vi "ScannerMain.vi"() -> ()   [LabVIEW 2012]
uses:
  Strict Type Def - Scan Parameters Cluster.ctl
  Strict Type Def - Optimize Parameters Cluster.ctl
  Rabi Window Parameters.ctl
  ESR Window Parameters.ctl
  Spin Echo Window Parameters.ctl
  Window Parameters-CPMG.ctl
  SaveContrastOptions.ctl
  Window Parameters-XY4.ctl
  States.ctl
  Global Vars.vi
  Channels.vi
panel:
  in  "Program":T1(tab)=enum."CPMG"
  in  "Z Voltage":dbl min=-10.0 max=10.0 step=0.1
  in  "Continuous":bool
  in  "Green Laser (low-T)":bool caption="Scan"
  in  "Microwave":bool caption="Scan"
  in  "Green Laser":bool=TRUE caption="Scan"
  out "Counts Intensity Graph":i32[][](graph)
  in  "Scan Parameters":T2={"X Max"=1.5, "X Min"=-1.5, "X Step"=0.02, "Y Max"=1.5, "Y Min"=-1.5, "Y Step"=0.02, "Dwell Time (ms) "=1} {"Dwell Time (ms)" min=0; "Y Step" min=0.0; "X Step" min=0.0}
  in  "Optimize":bool
  in  "Scan":bool
  in  "Count":bool caption="Optimize"
  out "Counts Chart":u32(graph)=11280
  out "Counts/s":i32=11280
  in  "Optimize Parameters":T3={"Volt Step"={"X"=0.005, "Y"=0.005, "Z"=0.0}, "Num Iterations"=5, "Dwell Time (ms)"=25, "Volts Range"={"X"=0.05, "Y"=0.05, "Z"=0.0}, "Method"={"X"=enum."Max", "Y"=enum."Max", "Z"=enum."Max"}} {"Volts Range"."Z" min=0.0; "Volts Range"."Y" min=0.0; "Volts Range"."X" min=0.0; "Dwell Time (ms)" min=0; "Num Iterations" min=1 step=1; "Volt Step"."Z" min=0.0; "Volt Step"."Y" min=1e-06; "Volt Step"."X" min=1e-06}
  in  "ESR":bool caption="Scan"
  in  "ESR spectrum spreadsheet":path=path "C:/experiment/data/may_15_2012/SIL1_NV1_pippin_uW_off"
  in  "Save ESR spectrum data":bool
  in  "ESR spectrum graph":path=path "C:/experiment/data/may_15_2012/SIL1_NV1_pippin_uW_off"
  in  "Save ESR spectrum graph":bool
  out "Avg ESR spectrum":cluster{"Y":dbl[], "Y":dbl[]}[](graph)=[{"Y"=[2.82, 2.8202499999999997, 2.8205, 2.82075, 2.8209999999999997, 2.82125, 2.8215, 2.8217499999999998, 2.822, 2.82225, 2.8225, 2.8227499999999996, 2.823, 2.82325, 2.8234999999999997, 2.82375, 2.824, 2.8242499999999997, 2.8245, 2.82475, 2.8249999999999997, 2.82525, 2.8255, 2.8257499999999998, 2.8259999999999996, 2.82625, 2.8265, 2.8267499999999997, 2.827, 2.82725, 2.8274999999999997, 2.82775, 2.828, 2.8282499999999997, 2.8285, 2.82875, 2.8289999999999997, 2.82925, 2.8295, 2.8297499999999998, 2.83, 2.83025, 2.8305, 2.8307499999999997, 2.831, 2.83125, 2.8314999999999997, 2.83175, 2.832, 2.8322499999999997, 2.8325, 2.83275, 2.8329999999999997, 2.83325, 2.8335, 2.8337499999999998, 2.8339999999999996, 2.83425, 2.8345, 2.8347499999999997, 2.835, 2.83525, 2.8354999999999997, 2.83575, 2.836, 2.8362499999999997, 2.8365, 2.83675, 2.8369999999999997, 2.83725, 2.8375, 2.8377499999999998, 2.838, 2.83825, 2.8385, 2.8387499999999997, 2.839, 2.83925, 2.8394999999999997, 2.83975, 2.84], "Y"=[256.4611111111111, 260.3277777777778, 260.22777777777776, 259.8, 256.4, 257.15, 255.9388888888889, 257.1111111111111, 259.4166666666667, 256.89444444444445, 256.6111111111111, 257.1333333333333, 258.4611111111111, 257.9222222222222, 256.1333333333333, 256.74444444444447, 255.5388888888889, 257.95, 255.46666666666667, 254.41666666666666, 255.3, 253.4611111111111, 253.63888888888889, 255.43333333333334, 252.68333333333334, 250.01111111111112, 248.7722222222222, 249.03333333333333, 247.25, 249.34444444444443, 248.07222222222222, 248.8, 250.05, 251.64444444444445, 250.7, 252.01111111111112, 248.62222222222223, 251.03333333333333, 248.46666666666667, 249.4388888888889, 249.24444444444444, 248.97222222222223, 250.43333333333334, 250.25, 252.8388888888889, 253.66666666666666, 253.85555555555555, 253.97222222222223, 257.25, 256.47777777777776, 257.18333333333334, 257.6722222222222, 257.19444444444446, 257.81111111111113, 257.4555555555556, 256.5444444444444, 260.69444444444446, 257.3722222222222, 258.3, 259.3722222222222, 258.1611111111111, 259.81666666666666, 258.8333333333333, 257.68333333333334, 255.70555555555555, 260.22222222222223, 256.3777777777778, 258.59444444444443, 260.6666666666667, 257.40555555555557, 257.5833333333333, 259.4555555555556, 259.5777777777778, 259.68888888888887, 258.97222222222223, 258.35, 258.84444444444443, 258.34444444444443, 260.6333333333333, 256.51666666666665, 259.43333333333334]}]
  out "Counts vs. frequency":i32[][](graph)
  in  "# freq points":i32=81
  in  "MW start freq (GHz)":dbl=2.82
  in  "MW stop freq (GHz)":dbl=2.84
  in  "# scans before track":i32=20
  in  "#scan iterations":i32=20
  in  "ESR Parameters":T4={"Window 1 time (s)"=0.005, "Window 2 time (s)"=5e-06, "Window 3 time (s) "=0.02, "Window 4 time (s)"=5e-07, "Window 4 channels"=[TRUE, FALSE, FALSE, TRUE], "Window 3 channels"=[TRUE, FALSE, TRUE, TRUE], "Window 2 channels"=[TRUE, FALSE, FALSE, TRUE], "Window 1 channels"=[TRUE, TRUE, FALSE, TRUE], "Path to ESR Burner"=path "C:/Users/Loncar/Desktop/ESR VIs - Srujan/Sam Kim/PB/ESRFreq.exe"}
  out "Rabi # scans done":u32=3
  in  "Save Rabi Contrast Options":T5={"Save contrast graph"=TRUE, "Path for contrast graph"=path "C:/Users/Public/Documents/Srujan/2014-06-22/NV3_Rabi_2p83GHz_3dBm_.jpg", "Save contrast data"=TRUE, "Path for contrast data"=path "C:/Users/Public/Documents/Srujan/2014-06-22/NV3_Rabi_2p83GHz_3dBm.txt"}
  in  "# scan iterations":i32=100
  in  "Rabi Parameters":T6={"Window 1 time (s)"=3e-06, "Window 2 time (s)"=1e-06, "Window 3 min time (s) "=1.2e-08, "Window 3 max time (s)"=3e-07, "Window 4 time (s)"=7.5e-07, "Window 5 time (s)"=3e-07, "Window 6 time (s)"=3e-06, "Window 7 time (s)"=3e-07, "Window 8 time (s)"=1e-07, "# samples before track"=100000, "# time axis points"=88, "Window 1 active channels"=[FALSE, FALSE, FALSE, TRUE], "Window 2 active channels"=[], "Window 3 active channels"=[TRUE], "Window 4 active channels"=[FALSE, FALSE, FALSE, TRUE], "Window 5 active channels "=[FALSE, FALSE, TRUE, TRUE], "Window 6 active channels"=[FALSE, FALSE, FALSE, TRUE], "Window 7 active channels"=[FALSE, FALSE, TRUE, TRUE], "Window 8 active channels"=[], "Path to Rabi Burner"=path "C:/Users/Loncar/Desktop/ESR VIs - Srujan/Sam Kim/PB/RabiBurn.exe"}
  out "Rabi Normalized contrast":cluster{"Y":dbl[], "Y":dbl[]}[](graph)=[{"Y"=[0.012, 0.015310344827586206, 0.018620689655172412, 0.02193103448275862, 0.025241379310344828, 0.02855172413793103, 0.031862068965517236, 0.035172413793103444, 0.03848275862068965, 0.04179310344827586, 0.04510344827586207, 0.048413793103448274, 0.05172413793103448, 0.05503448275862069, 0.0583448275862069, 0.0616551724137931, 0.0649655172413793, 0.0682758620689655, 0.07158620689655172, 0.07489655172413792, 0.07820689655172414, 0.08151724137931034, 0.08482758620689655, 0.08813793103448275, 0.09144827586206897, 0.09475862068965517, 0.09806896551724138, 0.10137931034482758, 0.1046896551724138, 0.108, 0.11131034482758621, 0.11462068965517241, 0.11793103448275863, 0.12124137931034482, 0.12455172413793103, 0.12786206896551724, 0.13117241379310343, 0.13448275862068965, 0.13779310344827586, 0.14110344827586205, 0.14441379310344826, 0.14772413793103448, 0.1510344827586207, 0.15434482758620688, 0.1576551724137931, 0.1609655172413793, 0.16427586206896552, 0.1675862068965517, 0.17089655172413792, 0.17420689655172414, 0.17751724137931035, 0.18082758620689654, 0.18413793103448275, 0.18744827586206897, 0.19075862068965518, 0.19406896551724137, 0.19737931034482759, 0.2006896551724138, 0.204, 0.2073103448275862, 0.21062068965517242, 0.21393103448275863, 0.21724137931034482, 0.22055172413793103, 0.22386206896551725, 0.22717241379310346, 0.23048275862068965, 0.23379310344827586, 0.23710344827586208, 0.24041379310344826, 0.24372413793103445, 0.24703448275862067, 0.25034482758620685, 0.2536551724137931, 0.2569655172413793, 0.2602758620689655, 0.2635862068965517, 0.2668965517241379, 0.27020689655172414, 0.2735172413793103, 0.2768275862068965, 0.28013793103448276, 0.28344827586206894, 0.28675862068965513, 0.2900689655172414, 0.29337931034482756, 0.2966896551724138, 0.3], "Y"=[-0.04069329314242657, -0.09175627240143368, -0.10250737463126836, -0.1041369472182596, -0.1326530612244897, -0.17416131334760881, -0.21134751773049645, -0.28631284916201116, -0.2211336599020295, -0.23330887747615559, -0.24717514124293793, -0.15837796480489677, -0.2288888888888888, -0.19809244314013202, -0.22746781115879822, -0.2178289000718907, -0.24873463485177152, -0.19629629629629627, -0.22723908216136196, -0.18337218337218333, -0.22245762711864406, -0.21386861313868616, -0.19219440353460968, -0.15828402366863914, -0.17686072218128232, -0.1615720524017467, -0.1755780346820809, -0.16607773851590105, -0.17273376159885798, -0.17988668555240797, -0.08751902587519025, -0.144561403508772, -0.10611643330876937, -0.05519244734930999, -0.0967741935483871, -0.08202567760342368, -0.05878030859662016, -0.11530398322851156, -0.02666666666666661, -0.05982905982905986, -0.0817790530846484, -0.06971830985915502, -0.024630541871921156, 0.014136904761904701, 0.0014609203798392392, 0.03252032520325199, -0.012587412587412559, 0.030124908155767738, 0.013148283418553659, 0.0806451612903226, 0.013768115942029053, 0.06661786237188867, 0.05203619909502273, -0.03856749311294764, -0.0029651593773165385, 0.019636363636363594, 0.00670141474311255, -0.021276595744680875, 0.004360465116279144, 0.024924471299093687, -0.08573436401967666, -0.05029154518950435, -0.02552881108679793, -0.0648148148148149, -0.10436713545521835, -0.09770114942528736, -0.05377147124719941, -0.13543859649122814, -0.11997019374068557, -0.16049382716049373, -0.10194902548725639, -0.13120830244625653, -0.161504424778761, -0.1736311239193084, -0.18084345961401008, -0.21134020618556695, -0.22222222222222218, -0.2334047109207709, -0.2154065620542083, -0.25215517241379304, -0.15744680851063828, -0.2404795486600846, -0.24043321299638987, -0.1862955032119914, -0.20865862313697658, -0.22429906542056083, -0.19926739926739928, -0.2138769670958512]}]
  in  "Rabi":bool caption="Scan"
  in  "Rabi Pause":bool
  out "SpinEcho scans done":u32=88
  in  "Pause Spin Echo":bool
  in  "SpinEcho Save Options":T5={"Save contrast graph"=TRUE, "Path for contrast graph"=path "C:/Users/Public/Documents/Srujan/2014-06-22/NV3_Echo_2p83GHz3dBm_pi64ns_150us.jpg", "Save contrast data"=TRUE, "Path for contrast data"=path "C:/Users/Public/Documents/Srujan/2014-06-22/NV3_Echo_2p83GHz3dBm_pi64ns_150us.txt"}
  in  "# SpinEcho scan iterations":i32=500
  in  "Spin Echo Parameters":T7={"Path to Spin Echo Burner"=path "C:/Users/Loncar/Desktop/ESR VIs - Srujan/Sam Kim/PB/SpinEchoBurn.exe", "Window 1 time (s)"=3e-06, "Window 1 active channels"=[FALSE, FALSE, FALSE, TRUE], "Window 10 time (s)"=3e-06, "Window 10 active channels"=[FALSE, FALSE, FALSE, TRUE], "# samples"=20000, "Window 2 time (s)"=1e-06, "Window 2 active channels"=[], "Window 4 min time (s) "=1.2e-08, "Window 4 active channels"=[FALSE], "Window 8 time (s)"=7.5e-07, "Window 8 active channels"=[FALSE, FALSE, FALSE, TRUE], "Window 9 time (s)"=3e-07, "Window 9 active channels "=[FALSE, FALSE, TRUE, TRUE], "# time axis points"=150, "Window 11 time (s)"=3e-07, "Window 11 active channels"=[FALSE, FALSE, TRUE, TRUE], "Window 12 time (s)"=1e-07, "Window 12 active channels"=[], "Window 4 max time (s)"=0.00015, "Window 3 time (s)"=3.2e-08, "Window 5 time (s)"=6.4e-08, "Window 3 active channels"=[TRUE, FALSE, FALSE, FALSE], "Window 5 active channels"=[TRUE, FALSE, FALSE, FALSE], "Window 7 time (s)"=3.2e-08, "Window 7 active channels"=[TRUE, FALSE, FALSE, FALSE]}
  out "Spin Echo contrast":cluster{"Y":dbl[], "Y":dbl[]}[](graph)=[{"Y"=[0.012, 1.0186308724832216, 2.025261744966443, 3.0318926174496648, 4.038523489932886, 5.045154362416107, 6.051785234899329, 7.058416107382551, 8.065046979865771, 9.071677852348992, 10.078308724832214, 11.084939597315435, 12.091570469798658, 13.098201342281879, 14.1048322147651, 15.111463087248321, 16.118093959731542, 17.124724832214763, 18.131355704697985, 19.137986577181206, 20.144617449664427, 21.151248322147648, 22.15787919463087, 23.164510067114094, 24.17114093959732, 25.17777181208054, 26.18440268456376, 27.191033557046982, 28.197664429530203, 29.204295302013424, 30.210926174496645, 31.217557046979863, 32.224187919463084, 33.23081879194631, 34.237449664429526, 35.244080536912755, 36.25071140939597, 37.2573422818792, 38.26397315436242, 39.27060402684564, 40.27723489932886, 41.28386577181208, 42.2904966442953, 43.297127516778524, 44.303758389261745, 45.310389261744966, 46.31702013422819, 47.32365100671141, 48.33028187919464, 49.33691275167785, 50.34354362416108, 51.35017449664429, 52.35680536912752, 53.363436241610735, 54.37006711409396, 55.37669798657718, 56.383328859060406, 57.38995973154362, 58.39659060402685, 59.40322147651006, 60.40985234899329, 61.41648322147651, 62.423114093959725, 63.42974496644295, 64.43637583892617, 65.4430067114094, 66.44963758389262, 67.45626845637584, 68.46289932885907, 69.46953020134228, 70.47616107382551, 71.48279194630872, 72.48942281879195, 73.49605369127516, 74.5026845637584, 75.50931543624161, 76.51594630872484, 77.52257718120805, 78.52920805369128, 79.53583892617449, 80.54246979865772, 81.54910067114093, 82.55573154362416, 83.56236241610739, 84.5689932885906, 85.57562416107382, 86.58225503355705, 87.58888590604028, 88.59551677852349, 89.6021476510067, 90.60877852348993, 91.61540939597316, 92.62204026845637, 93.6286711409396, 94.63530201342282, 95.64193288590604, 96.64856375838927, 97.65519463087249, 98.6618255033557, 99.66845637583893, 100.67508724832216, 101.68171812080537, 102.68834899328859, 103.69497986577181, 104.70161073825504, 105.70824161073826, 106.71487248322147, 107.7215033557047, 108.72813422818793, 109.73476510067114, 110.74139597315435, 111.74802684563758, 112.75465771812081, 113.76128859060404, 114.76791946308724, 115.77455033557047, 116.7811812080537, 117.78781208053692, 118.79444295302014, 119.80107382550335, 120.80770469798658, 121.81433557046981, 122.82096644295304, 123.82759731543625, 124.83422818791945, 125.84085906040268, 126.8474899328859, 127.85412080536912, 128.86075167785236, 129.86738255033558, 130.8740134228188, 131.88064429530203, 132.88727516778525, 133.89390604026843, 134.90053691275168, 135.9071677852349, 136.91379865771813, 137.92042953020135, 138.92706040268456, 139.9336912751678, 140.94032214765102, 141.9469530201342, 142.95358389261744, 143.96021476510066, 144.9668456375839, 145.97347651006712, 146.98010738255033, 147.98673825503357, 148.9933691275168, 150.0], "Y"=[-0.001288106483469231, -0.10181043663471774, -0.10525227460711332, -0.1414120126448893, -0.16048606746281158, -0.15417017691659646, -0.17425531914893608, -0.135445460344461, -0.13563267033432075, -0.14603378233910627, -0.11709956709956706, -0.1279896574014222, -0.09371554575523704, -0.1451820128479657, -0.1382219338092148, -0.12380952380952383, -0.1492152225327886, -0.13170212765957437, -0.13457424047924685, -0.12949181373591326, -0.10309278350515458, -0.14182436742504784, -0.08152894387980554, -0.1417862497322767, -0.10333622183708828, -0.10199220441749686, -0.14182128385583284, -0.12165345898479338, -0.15010570824524305, -0.11865509761388293, -0.16673828964331758, -0.11666666666666682, -0.16012861736334397, -0.17975206611570255, -0.16109229466553776, -0.12210435159125348, -0.1308674021198355, -0.14204425711275026, -0.1100352112676055, -0.1136214082035534, -0.14795160263213752, -0.09138724523339899, -0.10274423710208569, -0.11333617383894332, -0.07573112178088177, -0.12045357295678209, -0.08095238095238094, -0.09143593045717971, -0.13096511876738717, -0.12619098030912548, -0.16011829319814114, -0.14911903738719376, -0.1376578891029759, -0.13912671232876708, -0.14261094355881085, -0.1510867271576282, -0.14218716691536987, -0.14075630252100832, -0.13527508090614884, -0.11606571367612548, -0.15700534759358287, -0.12217001281503634, -0.1477707006369426, -0.15515409139213607, -0.13235916984328674, -0.10653070080277707, -0.1522853481418197, -0.1416021752771386, -0.12825948696205222, -0.16774597869229171, -0.17075232459847856, -0.1259211096662332, -0.1443364327979714, -0.11520837879118484, -0.1219081272084805, -0.1441750697275263, -0.15758091993185697, -0.12407488027862434, -0.15174182517631965, -0.16741309447643418, -0.15785001062247714, -0.15221124946328898, -0.14595283620140212, -0.15093941313067338, -0.1531932951410992, -0.13467230443974618, -0.16297234536626545, -0.16240953597275426, -0.14736387208297314, -0.1227659574468084, -0.1275728987993139, -0.11125683060109291, -0.10440985732814524, -0.1789251844046365, -0.14576198630136988, -0.11412205331570828, -0.12855614973262025, -0.16673640167364015, -0.1642993428026287, -0.12225772097976573, -0.13460712752254184, -0.13096774193548388, -0.11907894736842116, -0.10938883968113369, -0.13653056815726938, -0.16673562267273492, -0.14321926489226883, -0.17205444491705646, -0.13900955690703742, -0.14501703577512778, -0.11769872639437852, -0.140320485058467, -0.13874788494077825, -0.14436026936026938, -0.13037865748709135, -0.11130434782608685, -0.10467166152490091, -0.12107329842931935, -0.1390076988879385, -0.14327855035819634, -0.15853915980578412, -0.10110375275938176, -0.13623005877413943, -0.13019271948608133, -0.15475687103594082, -0.14588634435962683, -0.10822417865578697, -0.1448648648648649, -0.1680672268907562, -0.10934089917066776, -0.12374438982688596, -0.1423404255319149, -0.1595942868971227, -0.15227792802163512, -0.11069624423457075, -0.14535007448393272, -0.13879384088964933, -0.14793281653746765, -0.15410245730945432, -0.13261192446424783, -0.131000640068274, -0.13060344827586204, -0.14500941619585675, -0.11890963726121492, -0.10711938663745885, -0.13460303873314783, -0.1521467278032514, -0.17223161453930697, -0.16698212407991597, -0.13097039118219145]}]
  in  "Spin Echo":bool caption="Scan"
  out "CPMG scans done":u32=88
  in  "Save CPMG Contrast Options":T5={"Save contrast graph"=TRUE, "Path for contrast graph"=path "C:/Users/Public/Documents/Srujan/2014-06-22/NV3_CPMG_n2_2p83GHz3dBm_pi64ns_100us.jpg", "Save contrast data"=TRUE, "Path for contrast data"=path "C:/Users/Public/Documents/Srujan/2014-06-22/NV3_CPMG_n2_2p83GHz3dBm_pi64ns_100us.txt"}
  out "CPMG contrast":cluster{"Y":dbl[], "Y":dbl[]}[](graph)
  in  "CPMG":bool=TRUE caption="Scan"
  in  "# scan iterations":i32=200
  in  "CPMG Parameters":T8={"Path to CPMG Burner"=path "C:/Users/Loncar/Desktop/ESR VIs - Srujan/Sam Kim/PB/SpinEchoBurn.exe", "Window 1 time (s)"=3e-06, "Window 1 active channels"=[FALSE, FALSE, FALSE, TRUE], "Window 10 time (s)"=3e-06, "Window 10 active channels"=[FALSE, FALSE, FALSE, TRUE], "Window 2 time (s)"=1e-06, "Window 2 active channels"=[], "Window 4 min time (s) "=1.2e-08, "Window 4 active channels"=[FALSE], "Window 8 time (s)"=7.5e-07, "Window 8 active channels"=[FALSE, FALSE, FALSE, TRUE], "Window 9 time (s)"=3e-07, "Window 9 active channels "=[FALSE, FALSE, TRUE, TRUE], "# delay time points"=100, "Window 11 time (s)"=3e-07, "Window 11 active channels"=[FALSE, FALSE, TRUE, TRUE], "Window 12 time (s)"=1e-07, "Window 12 active channels"=[], "Window 4 max time (s)"=0.0001, "Window 3 time (s)"=3.2e-08, "Window 5 time (s)"=6.4e-08, "Window 3 active channels"=[TRUE, FALSE, FALSE, FALSE], "Window 5 active channels"=[TRUE, FALSE, FALSE, FALSE], "# pi pulses"=2, "# samples before track"=20000} {"# pi pulses" min=1; "# delay time points" min=2}
  in  "Save XY-4 Contrast Options":T5={"Save contrast graph"=FALSE, "Path for contrast graph"=path "C:/experiment/data/may_15_2012/SIL1_NV1_pippin_uW_off", "Save contrast data"=FALSE, "Path for contrast data"=path "C:/experiment/data/may_15_2012/SIL1_NV1_pippin_uW_off"}
  out "XY-4 Normalized contrast":cluster{"Y":dbl[], "Y":dbl[]}[](graph)
  in  "XY-4":bool caption="Scan"
  in  "# scan iterations":i32
  in  "XY-4 Parameters":T9={"Path to CPMG Burner"=path "C:/Users/Loncar/Desktop/ESR VIs - Srujan/Sam Kim/PB/SpinEchoBurn.exe", "Window 1 time (s)"=3e-06, "Window 1 active channels"=[FALSE, FALSE, FALSE, TRUE], "Window 10 time (s)"=3e-06, "Window 10 active channels"=[FALSE, FALSE, FALSE, TRUE], "Window 2 time (s)"=0.0, "Window 2 active channels"=[], "Window 4 min time (s) "=0.0, "Window 4 active channels"=[FALSE], "Window 8 time (s)"=7.5e-07, "Window 8 active channels"=[FALSE, FALSE, FALSE, TRUE], "Window 9 time (s)"=2e-07, "Window 9 active channels "=[FALSE, FALSE, TRUE, TRUE], "# time points"=2, "Window 11 time (s)"=0.0, "Window 11 active channels"=[FALSE, FALSE, TRUE, TRUE], "Window 12 time (s)"=1e-07, "Window 12 active channels"=[], "Window 4 max time (s)"=0.0, "Window 3 time (s)"=0.0, "Window 5 time (s)"=5e-06, "Window 3 active channels"=[TRUE, FALSE, FALSE, FALSE], "Window 5c active channels"=[TRUE, FALSE, FALSE, FALSE], "# pulse sequences"=1, "# samples before track"=0, "Window 5a active channels"=[TRUE, FALSE, FALSE, FALSE]} {"# pulse sequences" min=1; "# time points" min=2}
  in  "Z AO Channel":tag="Dev1/ao3"
  in  "Laser voltage":tag="Dev1/ao2"
  in  "Counter(s)":tag="Dev1/ctr0"
  in  "X AO Channel":tag="Dev1/ao0"
  in  "Y AO Channel":tag="Dev1/ao1"
  in  "Sample clock line":tag="/Dev1/PFI9"
  in  "spinapi.dll":path=path "C:/SpinCore/SpinAPI/dll/spinapi64.dll"
  in  "HoldChannel.exe":path=path "C:/Users/Loncar/Desktop/ESR VIs - Srujan/Sam Kim/PB/HoldChannel.exe"
  # "Note for Z: 1 V = 10 um"
  # "Z tracking does NOT work!!!!"
  # "X, Y, and Z display values\nonly update after manual\noptimization"
  # "Default PB connections:\nPB0 - MW switch\nPB3 - Green AOM\n\nDefault for low-T:\nPB1 - Green AOM"
  # "ESR spectrum measurement"
  # "Default PB connections:\nPB0 - MW switch\nPB1 - MW freq step\nPB2 - Counter sample clk\nPB3 - Green AOM"
  # "Pulse sequence parameters - Window durations and PB channel states"
  # "Green AOM, MW switch are always on!"
  # "(to spreadsheet)"
  # "MW freq step\ndwell time"
  # "MW freq step"
  # "Wait"
  # "Fluorescence\ncounting"
  # "Ctr sample clk"
  # "Wait"
  # "Rabi measurement"
  # "Default PB connections:\nPB0 - MW switch\nPB1 - unused\nPB2 - Counter sample clk\nPB3 - Green AOM"
  # "to spreadsheet"
  # "Initialization"
  # "Green AOM"
  # "Wait"
  # "All off"
  # "MW pulsing"
  # "MW"
  # "Wait"
  # "Green AOM"
  # "Green AOM,\ncounter clk"
  # "Readout"
  # "Repump"
  # "Green AOM"
  # "Green AOM,\ncounter clk"
  # "Reference"
  # "All off"
  # "Wait (nominal)"
  # "Spin Echo measurement"
  # "Default PB connections:\nPB0 - MW switch\nPB1 - unused\nPB2 - Counter sample clk\nPB3 - Green AOM"
  # "to spreadsheet"
  # "Green AOM"
  # "Initialization"
  # "All off"
  # "Wait"
  # "MW"
  # "MW pulse 1"
  # "All off"
  # "Free precession 1"
  # "max: ~350"
  # "MW pulse 2"
  # "MW"
  # "Free precession 2: Window 6"
  # "MW"
  # "MW pulse 1"
  # "Green AOM"
  # "Wait"
  # "Green AOM,\ncounter clk"
  # "Readout"
  # "Green AOM"
  # "Repump"
  # "Green AOM,\ncounter clk"
  # "Reference"
  # "Wait (nominal)"
  # "All off"
  # "CPMG measurement"
  # "Default PB connections:\nPB0 - MW switch\nPB1 - MW 90deg phase shifted\nPB2 - Counter sample clk\nPB3 - Green AOM"
  # "to spreadsheet"
  # "Green AOM"
  # "Initialization"
  # "All off"
  # "Wait"
  # "MW pulse 1\n(pi/2)"
  # "MW"
  # "Free precession\n(Tau/2)"
  # "All off"
  # "max: ~350"
  # "MW pulse 2\n(pi90)"
  # "MW90"
  # "Free precession (Tau/2)\nMW pulse 1 (pi/2)"
  # "Window 6 = Window 4\nWindow 7 = Window 3"
  # "All off\nMW"
  # "Green AOM"
  # "Wait for green"
  # "Green AOM,\ncounter clk"
  # "Readout"
  # "Green AOM"
  # "Repump"
  # "Green AOM,\ncounter clk"
  # "Reference"
  # "Wait (nominal)"
  # "All off"
  # "XY-4 measurement"
  # "Default PB connections:\nPB0 - MW switch\nPB1 - MW 90deg phase shifted\nPB2 - Counter sample clk\nPB3 - Green AOM"
  # "to spreadsheet"
  # "pulse=XYXY"
  # "max: ~350"
  # "x 4=#pi pulses"
  # "Green AOM"
  # "Initialization"
  # "All off"
  # "Wait"
  # "MW pulse 1\n(pi/2)"
  # "MW"
  # "Free precession\n(T/2)"
  # "All off"
  # "MW (X)"
  # "MW pulse 2\n(pi)"
  # "MW90 (Y)"
  # "Pulse Sequence=[T/2-Pi-T-Pi90-T-Pi-T-Pi90-T/2]^N\nMW pulse 1 (pi/2)"
  # "Window 4-5a-g-6\nWindow 7"
  # "Green AOM"
  # "Wait for green"
  # "Green AOM,\ncounter sample clk"
  # "Readout"
  # "Green AOM"
  # "Repump"
  # "Green AOM,\ncounter sample clk"
  # "Reference"
  # "Wait (nominal)"
  # "All off"
  # "TODO:\nHigh priority:\nShow counts during pulsed experiments\n\nMedium priority:\nChanges in Srujan's low-T experiments\n\nLow priority:\nContinuous Scan does not save image\nSave Counts Intensity Graph as image to clipbard\nAllow ESR+pulsed experiments to stop and save\n    (1. Stop at end of run; 2. Force stop)\nImplement new tracking algorithm for noisy data\n    (Ensemble NV centers)\nAllow stopping in middle of optimize\nAllow count concurrently with optimize/scan(?)"
  # "Author: Samuel Kim\nESR, Rabi, and Spin Echo experiments adapted from Srujan"
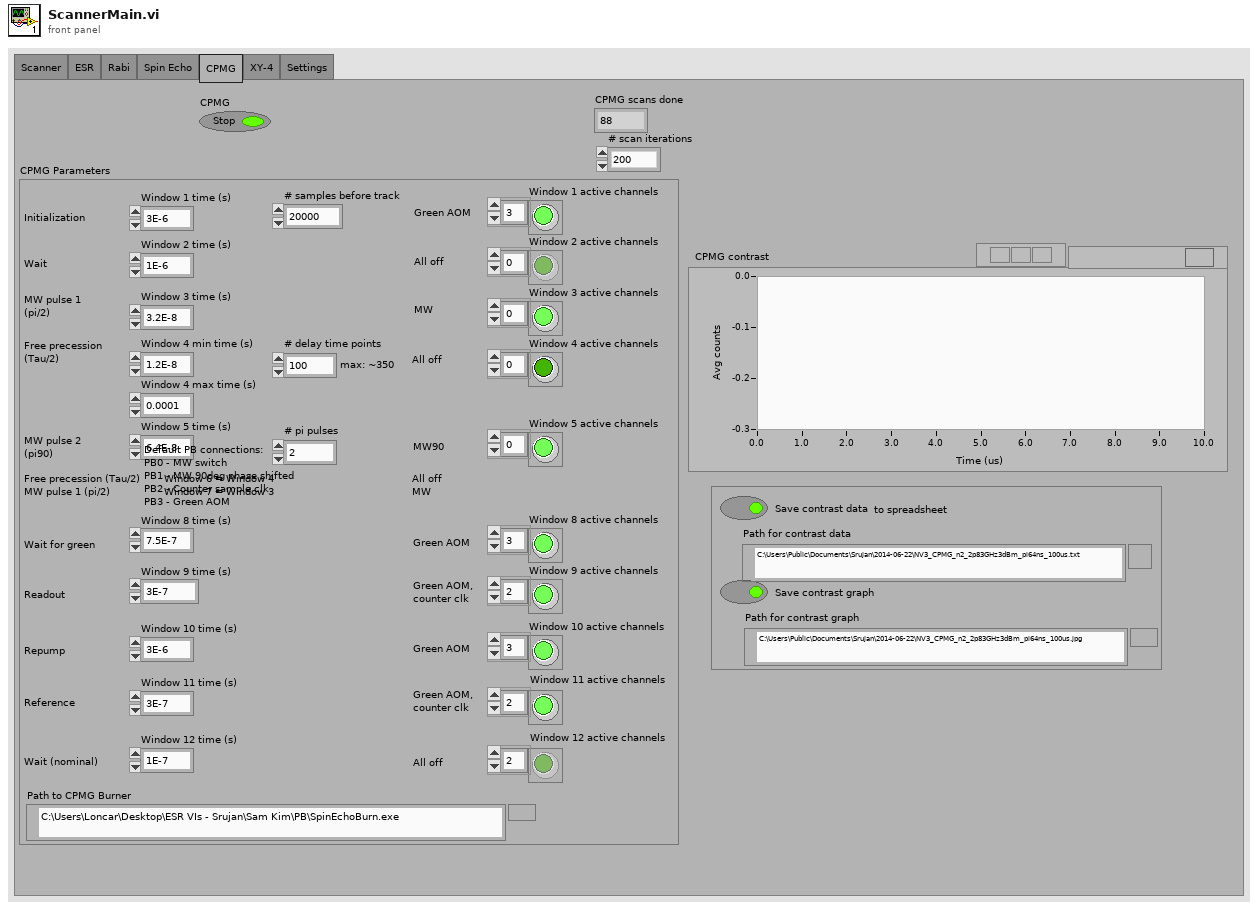
[diagram p1: front panel]
types:
  T1 = enum32{"Scanner", "ESR", "Rabi", "Spin Echo", "CPMG", "XY-4", "Settings"}
  T2 = typedef "Strict Type Def - Scan Parameters Cluster.ctl" = cluster{"X Max":dbl, "X Min":dbl, "X Step":dbl, "Y Max":dbl, "Y Min":dbl, "Y Step":dbl, "Dwell Time (ms) ":i32}
  T3 = typedef "Strict Type Def - Optimize Parameters Cluster.ctl" = cluster{"Volt Step":cluster{"X":dbl, "Y":dbl, "Z":dbl}, "Num Iterations":i32, "Dwell Time (ms)":i32, "Volts Range":cluster{"X":dbl, "Y":dbl, "Z":dbl}, "Method":cluster{"X":enum16{"Max", "Gaussian"}, "Y":enum16{"Max", "Gaussian"}, "Z":enum16{"Max", "Gaussian"}}}
  T4 = typedef "ESR Window Parameters.ctl" = cluster{"Window 1 time (s)":dbl, "Window 2 time (s)":dbl, "Window 3 time (s) ":dbl, "Window 4 time (s)":dbl, "Window 4 channels":bool[], "Window 3 channels":bool[], "Window 2 channels":bool[], "Window 1 channels":bool[], "Path to ESR Burner":path}
  T5 = typedef "SaveContrastOptions.ctl" = cluster{"Save contrast graph":bool, "Path for contrast graph":path, "Save contrast data":bool, "Path for contrast data":path}
  T6 = typedef "Rabi Window Parameters.ctl" = cluster{"Window 1 time (s)":dbl, "Window 2 time (s)":dbl, "Window 3 min time (s) ":dbl, "Window 3 max time (s)":dbl, "Window 4 time (s)":dbl, "Window 5 time (s)":dbl, "Window 6 time (s)":dbl, "Window 7 time (s)":dbl, "Window 8 time (s)":dbl, "# samples before track":i32, "# time axis points":i32, "Window 1 active channels":bool[], "Window 2 active channels":bool[], "Window 3 active channels":bool[], "Window 4 active channels":bool[], "Window 5 active channels ":bool[], "Window 6 active channels":bool[], "Window 7 active channels":bool[], "Window 8 active channels":bool[], "Path to Rabi Burner":path}
  T7 = typedef "Spin Echo Window Parameters.ctl" = cluster{"Path to Spin Echo Burner":path, "Window 1 time (s)":dbl, "Window 1 active channels":bool[], "Window 10 time (s)":dbl, "Window 10 active channels":bool[], "# samples":i32, "Window 2 time (s)":dbl, "Window 2 active channels":bool[], "Window 4 min time (s) ":dbl, "Window 4 active channels":bool[], "Window 8 time (s)":dbl, "Window 8 active channels":bool[], "Window 9 time (s)":dbl, "Window 9 active channels ":bool[], "# time axis points":i32, "Window 11 time (s)":dbl, "Window 11 active channels":bool[], "Window 12 time (s)":dbl, "Window 12 active channels":bool[], "Window 4 max time (s)":dbl, "Window 3 time (s)":dbl, "Window 5 time (s)":dbl, "Window 3 active channels":bool[], "Window 5 active channels":bool[], "Window 7 time (s)":dbl, "Window 7 active channels":bool[]}
  T8 = typedef "Window Parameters-CPMG.ctl" = cluster{"Path to CPMG Burner":path, "Window 1 time (s)":dbl, "Window 1 active channels":bool[], "Window 10 time (s)":dbl, "Window 10 active channels":bool[], "Window 2 time (s)":dbl, "Window 2 active channels":bool[], "Window 4 min time (s) ":dbl, "Window 4 active channels":bool[], "Window 8 time (s)":dbl, "Window 8 active channels":bool[], "Window 9 time (s)":dbl, "Window 9 active channels ":bool[], "# delay time points":i32, "Window 11 time (s)":dbl, "Window 11 active channels":bool[], "Window 12 time (s)":dbl, "Window 12 active channels":bool[], "Window 4 max time (s)":dbl, "Window 3 time (s)":dbl, "Window 5 time (s)":dbl, "Window 3 active channels":bool[], "Window 5 active channels":bool[], "# pi pulses":i32, "# samples before track":i32}
  T9 = typedef "Window Parameters-XY4.ctl" = cluster{"Path to CPMG Burner":path, "Window 1 time (s)":dbl, "Window 1 active channels":bool[], "Window 10 time (s)":dbl, "Window 10 active channels":bool[], "Window 2 time (s)":dbl, "Window 2 active channels":bool[], "Window 4 min time (s) ":dbl, "Window 4 active channels":bool[], "Window 8 time (s)":dbl, "Window 8 active channels":bool[], "Window 9 time (s)":dbl, "Window 9 active channels ":bool[], "# time points":i32, "Window 11 time (s)":dbl, "Window 11 active channels":bool[], "Window 12 time (s)":dbl, "Window 12 active channels":bool[], "Window 4 max time (s)":dbl, "Window 3 time (s)":dbl, "Window 5 time (s)":dbl, "Window 3 active channels":bool[], "Window 5c active channels":bool[], "# pulse sequences":i32, "# samples before track":i32, "Window 5a active channels":bool[]}
  T10 = typedef "States.ctl" = enum16{"Initialize", "Scan", "Count", "Optimize", "Hold", "ESR", "Rabi", "Spin Echo", "Spectrum", "Stability", "CPMG", "XY-4", "Exit"}
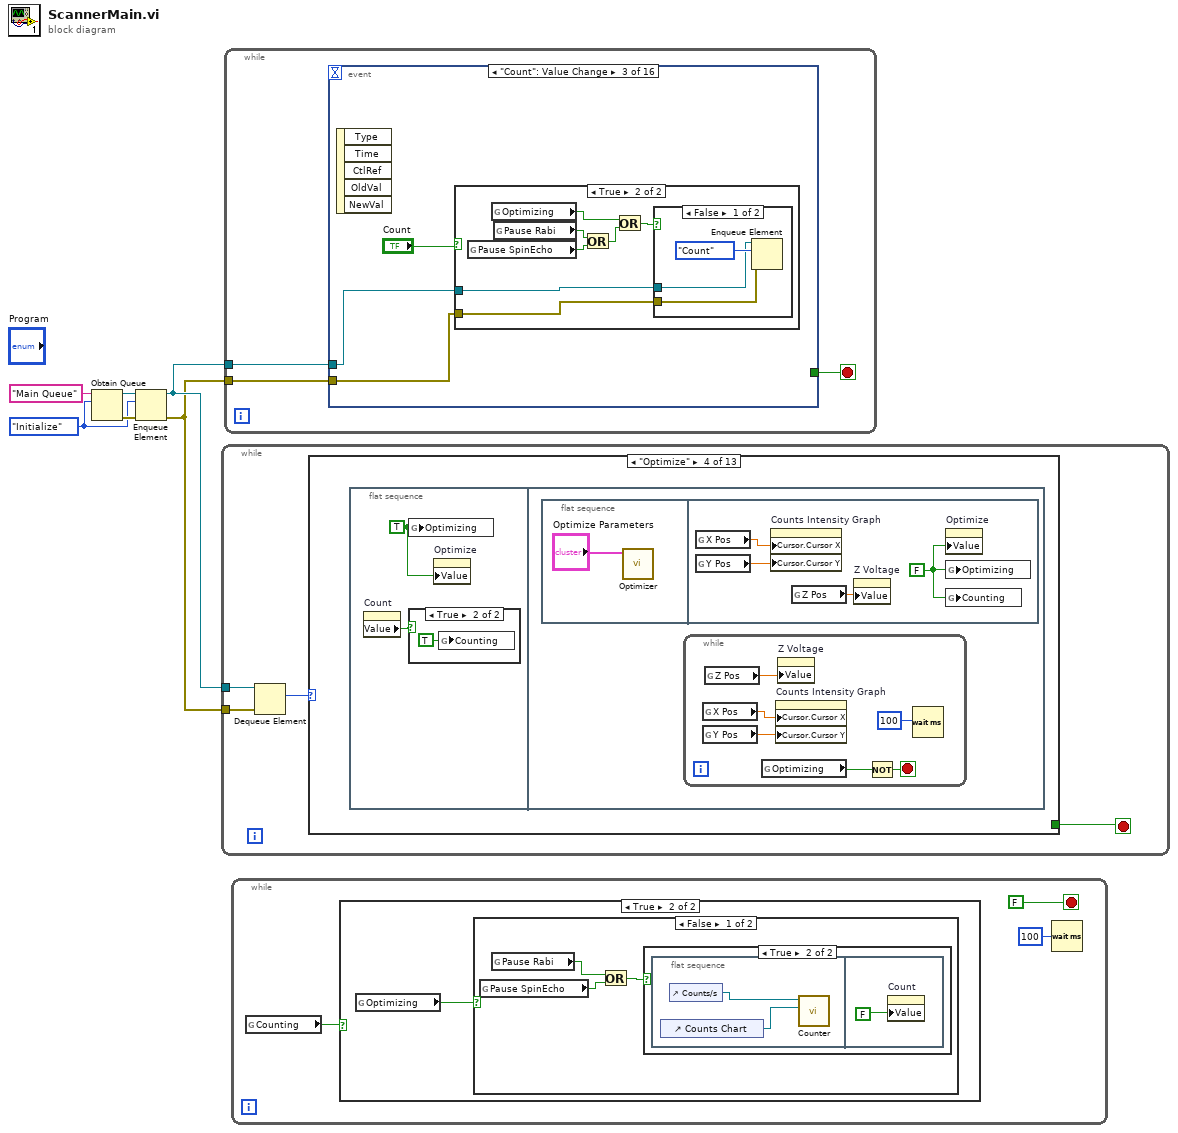
[diagram p0: block diagram]
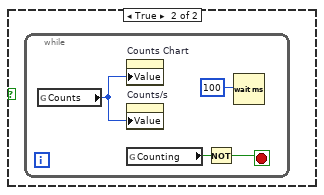
[diagram p4: hidden frame]
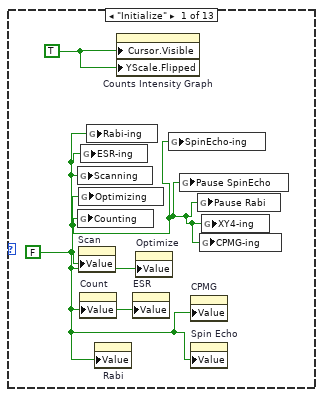
[diagram p5: hidden frame]
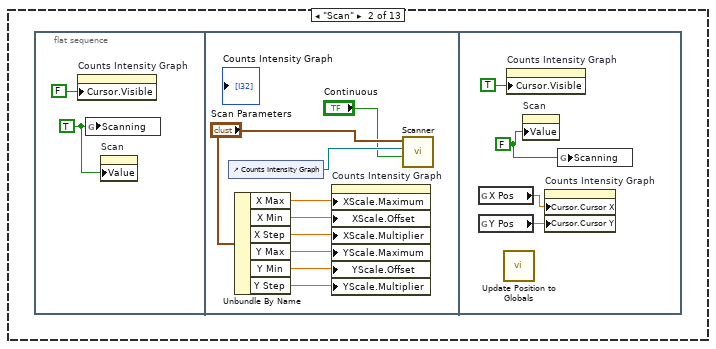
[diagram p6: hidden frame]
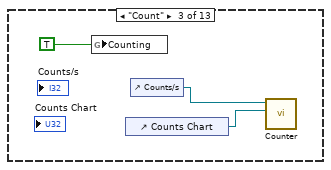
[diagram p7: hidden frame]
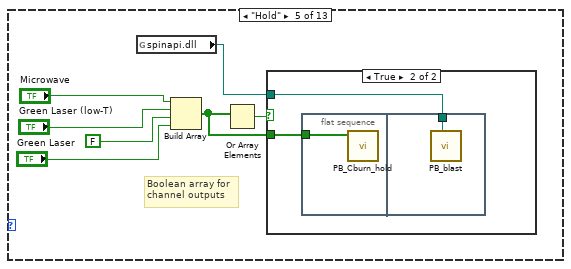
[diagram p9: hidden frame]
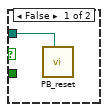
[diagram p10: hidden frame]
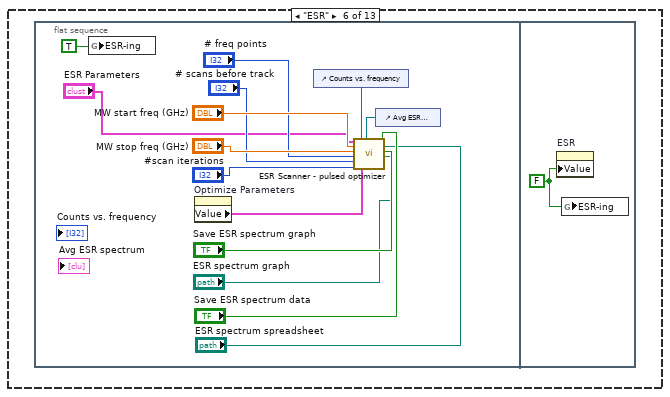
[diagram p11: hidden frame]
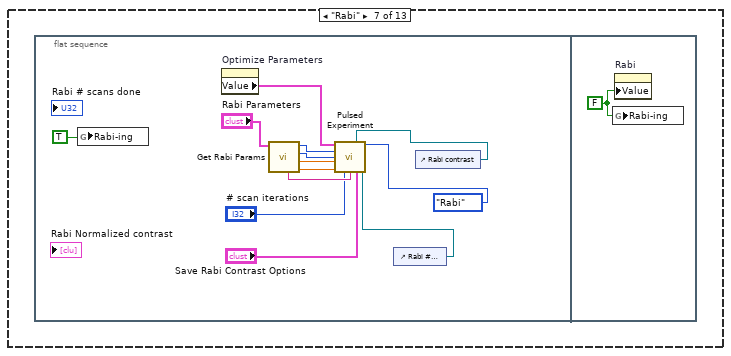
[diagram p12: hidden frame]
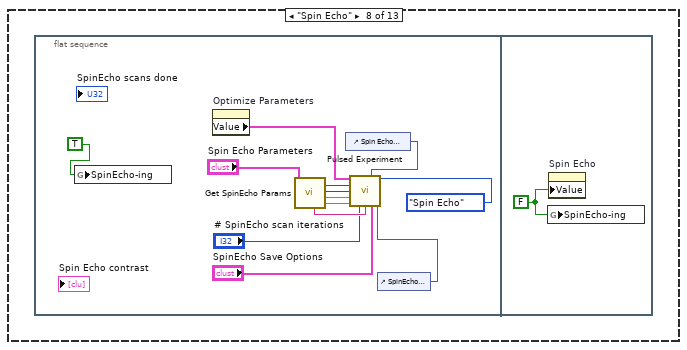
[diagram p13: hidden frame]
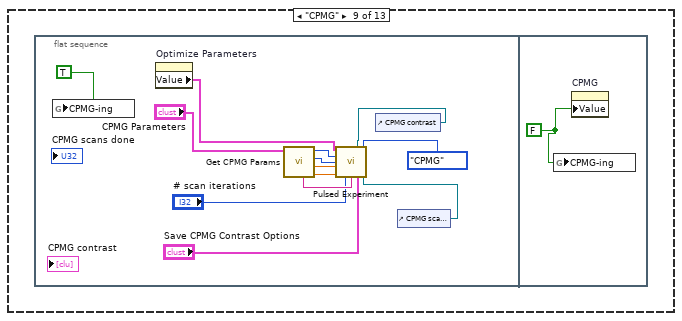
[diagram p14: hidden frame]
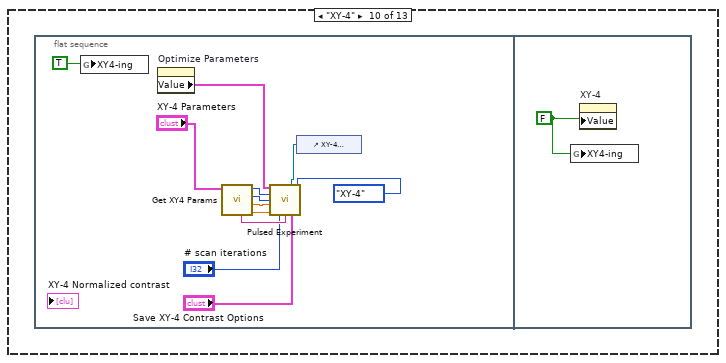
[diagram p15: hidden frame]
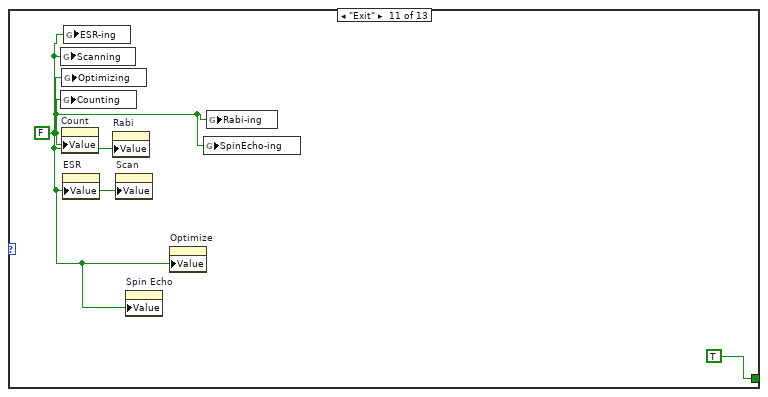
[diagram p16: hidden frame]
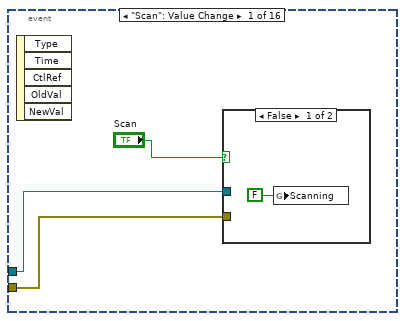
[diagram p19: hidden frame]
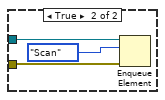
[diagram p20: hidden frame]
diagram:
  w1 = States."Initialize"
  n1 = Obtain Queue(name (unnamed)="Main Queue", element data type=w1) -> (queue out=w4:refnum<queue>, error out=w6:errorcluster)  [unwired: 3 in, 1 out]
  n2 = Enqueue Element(queue=w4, element=w1, error in (no error)=w6) -> (queue out=w3:refnum<queue>, error out=w2:errorcluster)  [unwired: 1 in, 1 out]
  n3 = while {
    tunnel: w3 -> [w9]
    tunnel: w2 -> [w8]
    stop <- w7 stop-if-true
    n4 = Dequeue Element(queue=w9, error in (no error)=w8) -> (element=w10:T10)  [unwired: 1 in, 3 out]
    n5 = case shown="\"Optimize\"" w10 {
      tunnel: [_ _ _ _ _ _ _ _ _ _ TRUE _ _] -> w7
      frame "Initialize" {
        w12 = TRUE
        w11 = FALSE
        n6 = global write "Global Vars.vi" "Scanning"(w11) -> ()
        n7 = global write "Global Vars.vi" "Counting"(w11) -> ()
        n8 = global write "Global Vars.vi" "Optimizing"(w11) -> ()
        n9 = property on="Scan" class="Bool (strict)"("Value"=w11) -> ()  [unwired: 2 in, 2 out]
        n10 = property on="Count" class="Bool (strict)"("Value"=w11) -> ()  [unwired: 2 in, 2 out]
        n11 = global write "Global Vars.vi" "ESR-ing"(w11) -> ()
        n12 = global write "Global Vars.vi" "Rabi-ing"(w11) -> ()
        n13 = property on="Rabi" class="Bool (strict)"("Value"=w11) -> ()  [unwired: 2 in, 2 out]
        n14 = property on="Counts Intensity Graph" class="IntGraph (strict)"("Cursor.Visible"=w12, "YScale.Flipped"=w12) -> ()  [unwired: 2 in, 2 out]
        n15 = property on="ESR" class="Bool (strict)"("Value"=w11) -> ()  [unwired: 2 in, 2 out]
        n16 = property on="Optimize" class="Bool (strict)"("Value"=w11) -> ()  [unwired: 2 in, 2 out]
        n17 = global write "Global Vars.vi" "SpinEcho-ing"(w11) -> ()
        n18 = global write "Global Vars.vi" "Pause SpinEcho"(w11) -> ()
        n19 = property on="CPMG" class="Bool (strict)"("Value"=w11) -> ()  [unwired: 2 in, 2 out]
        n20 = property on="Spin Echo" class="Bool (strict)"("Value"=w11) -> ()  [unwired: 2 in, 2 out]
        n21 = global write "Global Vars.vi" "Pause Rabi"(w11) -> ()
        n22 = global write "Global Vars.vi" "CPMG-ing"(w11) -> ()
        n23 = global write "Global Vars.vi" "XY4-ing"(w11) -> ()
      }
      frame "Scan" {
        n24 = flat-sequence {
          frame #0 {
            w13 = TRUE
            n25 = property on="Counts Intensity Graph" class="IntGraph (strict)"("Cursor.Visible"=FALSE) -> ()  [unwired: 2 in, 2 out]
            n26 = global write "Global Vars.vi" "Scanning"(w13) -> ()
            n27 = property on="Scan" class="Bool (strict)"("Value"=w13) -> ()  [unwired: 2 in, 2 out]
          }
          frame #1 {
            n28 = control-ref of="Counts Intensity Graph"() -> (w23:refnum<vi>)
            n29 = Unbundle By Name("Scan Parameters") -> ("X Max"=w18:dbl, "X Min"=w22:dbl, "X Step"=w21:dbl, "Y Max"=w20:dbl, "Y Min"=w19:dbl, "Y Step"=w16:dbl)
            n30 = property on="Counts Intensity Graph" class="IntGraph (strict)"("XScale.Maximum"=w18, "XScale.Offset"=w22, "XScale.Multiplier"=w21, "YScale.Maximum"=w20, "YScale.Offset"=w19, "YScale.Multiplier"=w16) -> ()  [unwired: 2 in, 2 out]
            n31 = call "Scanner.vi"("Continuous"="Continuous", "IntGraph Refnum"=w23, "Scan Parameters"="Scan Parameters") -> ()  [unwired: 8 in, 1 out]
          }
          frame #2 {
            w24 = FALSE
            n32 = global read "Global Vars.vi" "X Pos"() -> (w26:dbl)
            n33 = global read "Global Vars.vi" "Y Pos"() -> (w25:dbl)
            n34 = call "Update Position to Globals.vi"() -> ()  [unwired: 11 in, 1 out]
            n35 = property on="Counts Intensity Graph" class="IntGraph (strict)"("Cursor.Visible"=TRUE) -> ()  [unwired: 2 in, 2 out]
            n36 = property on="Scan" class="Bool (strict)"("Value"=w24) -> ()  [unwired: 2 in, 2 out]
            n37 = property on="Counts Intensity Graph" class="IntGraph (strict)"("Cursor.Cursor X"=w26, "Cursor.Cursor Y"=w25) -> ()  [unwired: 2 in, 2 out]
            n38 = global write "Global Vars.vi" "Scanning"(w24) -> ()
          }
        }
      }
      frame "Count" {
        n39 = global write "Global Vars.vi" "Counting"(TRUE) -> ()
        n40 = control-ref of="Counts Chart"() -> (w28:refnum<vi>)
        n41 = control-ref of="Counts/s"() -> (w29:refnum<vi>)
        n42 = call "Counter.vi"("Counts Chart Refnum"=w28, "Counts/s Ref"=w29) -> ()  [unwired: 10 in]
      }
      frame "Optimize" {
        n43 = flat-sequence {
          frame #0 {
            w32 = TRUE
            n44 = property on="Count" class="Bool (strict)"() -> ("Value"=w31:bool)  [unwired: 2 in, 2 out]
            n45 = global write "Global Vars.vi" "Optimizing"(w32) -> ()
            n46 = case shown="True" w31 {
              frame False {
              }
              frame True {
                n47 = global write "Global Vars.vi" "Counting"(TRUE) -> ()
              }
            }
            n48 = property on="Optimize" class="Bool (strict)"("Value"=w32) -> ()  [unwired: 2 in, 2 out]
          }
          frame #1 {
            n49 = flat-sequence {
              frame #0 {
                n50 = call "Optimizer.vi"("Optimize Parameters"="Optimize Parameters") -> ()  [unwired: 11 in]
              }
              frame #1 {
                w41 = FALSE
                n51 = global read "Global Vars.vi" "X Pos"() -> (w44:dbl)
                n52 = global read "Global Vars.vi" "Y Pos"() -> (w43:dbl)
                n53 = property on="Counts Intensity Graph" class="IntGraph (strict)"("Cursor.Cursor X"=w44, "Cursor.Cursor Y"=w43) -> ()  [unwired: 2 in, 2 out]
                n54 = global read "Global Vars.vi" "Z Pos"() -> (w42:dbl)
                n55 = property on="Z Voltage" class="DigNum (strict)"("Value"=w42) -> ()  [unwired: 2 in, 2 out]
                n56 = property on="Optimize" class="Bool (strict)"("Value"=w41) -> ()  [unwired: 2 in, 2 out]
                n57 = global write "Global Vars.vi" "Optimizing"(w41) -> ()
                n58 = global write "Global Vars.vi" "Counting"(w41) -> ()
              }
            }
            n59 = while {
              stop <- w39 stop-if-true
              n60 = global read "Global Vars.vi" "X Pos"() -> (w37:dbl)
              n61 = global read "Global Vars.vi" "Y Pos"() -> (w36:dbl)
              n62 = global read "Global Vars.vi" "Z Pos"() -> (w34:dbl)
              n63 = global read "Global Vars.vi" "Optimizing"() -> (w38:bool)
              n64 = property on="Counts Intensity Graph" class="IntGraph (strict)"("Cursor.Cursor X"=w37, "Cursor.Cursor Y"=w36) -> ()  [unwired: 2 in, 2 out]
              n65 = property on="Z Voltage" class="DigNum (strict)"("Value"=w34) -> ()  [unwired: 2 in, 2 out]
              n66 = Not(x=w38) -> (.not. x?=w39:bool)
              n67 = Wait (ms)(milliseconds to wait=u32 100 ("millisecond multiple")) -> ()  [unwired: 1 out]
            }
          }
        }
      }
      frame "Hold" {
        # "Boolean array for\nchannel outputs"
        n68 = global read "Channels.vi" "spinapi.dll"() -> (w51:path)
        n69 = Build Array("Microwave", "Green Laser (low-T)", FALSE, "Green Laser") -> (w45:bool[])
        n70 = Or Array Elements(Boolean array=w45) -> (logical OR=w50:bool)
        n71 = case shown="True" w50 {
          tunnel: w51 -> [w52 w54]
          tunnel: w45 -> [_ w53]
          frame False {
            n72 = call "PB_reset.vi"("Path to spinapi.dll"=w52) -> ()  [unwired: 7 in]
          }
          frame True {
            n73 = flat-sequence {
              tunnel: w53 -> [w55]
              tunnel: w54 -> [w56]
              frame #0 {
                n74 = call "PB_Cburn_hold.vi"("Optimize active channels"=w55) -> ()  [unwired: 9 in, 2 out]
              }
              frame #1 {
                n75 = call "PB_blast.vi"("Path to spinapi.dll"=w56) -> ()  [unwired: 7 in]
              }
            }
          }
        }
      }
      frame "ESR" {
        n76 = flat-sequence {
          frame #0 {
            n77 = global write "Global Vars.vi" "ESR-ing"(TRUE) -> ()
            n78 = property on="Optimize Parameters" class="Clust (strict)"() -> ("Value"=w61:T3)  [unwired: 2 in, 2 out]
            n79 = control-ref of="Counts vs. frequency"() -> (w63:refnum<vi>)
            n80 = control-ref of="Avg ESR spectrum"() -> (w62:refnum<vi>)
            n81 = call "ESR Scanner - pulsed optimizer.vi"("ESR Parameters"="ESR Parameters", "MW start freq (GHz)"="MW start freq (GHz)", "MW stop freq (GHz)"="MW stop freq (GHz)", "# freq points"="# freq points", "# scans before track"="# scans before track", "#scan iterations"="#scan iterations", "IntGraph Refnum"=w63, "Optimize Parameters"=w61, "XY Graph Refnum"=w62, "Save avg spectrum data to spreadsheet?"="Save ESR spectrum data", "Path for avg spectrum spreadsheet"="ESR spectrum spreadsheet", "Save avg spectrum graph?"="Save ESR spectrum graph", "Path for avg spectrum graph"="ESR spectrum graph") -> ()  [unwired: 7 in]
          }
          frame #1 {
            w71 = FALSE
            n82 = property on="ESR" class="Bool (strict)"("Value"=w71) -> ()  [unwired: 2 in, 2 out]
            n83 = global write "Global Vars.vi" "ESR-ing"(w71) -> ()
          }
        }
      }
      frame "Rabi" {
        n84 = flat-sequence {
          frame #0 {
            n85 = global write "Global Vars.vi" "Rabi-ing"(TRUE) -> ()
            n86 = property on="Optimize Parameters" class="Clust (strict)"() -> ("Value"=w77:T3)  [unwired: 2 in, 2 out]
            n87 = call "Get Rabi Params.vi"("Rabi Parameters"="Rabi Parameters") -> ("max time"=w80:dbl, "min time"=w81:dbl, "# time points"=w82:i32, "# samples"=w83:i32, "PB Window Args"=w79:string)  [unwired: 6 in]
            n88 = control-ref of="Rabi # scans done"() -> (w72:refnum<vi>)
            n89 = control-ref of="Rabi contrast"() -> (w74:refnum<vi>)
            n90 = call "Pulsed Experiment.vi"("Optimize Parameters"=w77, "Contrast XY Graph Refnum"=w74, "Experiment"=States."Rabi", "# samples"=w83, "# time points"=w82, "min time"=w81, "max time"=w80, "# scan iterations"="# scan iterations", "Window Parameters"=w79, "Save Contrast Options"="Save Rabi Contrast Options", "scans done ref"=w72) -> ()  [unwired: 5 in]
          }
          frame #1 {
            w85 = FALSE
            n91 = global write "Global Vars.vi" "Rabi-ing"(w85) -> ()
            n92 = property on="Rabi" class="Bool (strict)"("Value"=w85) -> ()  [unwired: 2 in, 2 out]
          }
        }
      }
      frame "Spin Echo" {
        n93 = flat-sequence {
          frame #0 {
            n94 = global write "Global Vars.vi" "SpinEcho-ing"(TRUE) -> ()
            n95 = property on="Optimize Parameters" class="Clust (strict)"() -> ("Value"=w96:T3)  [unwired: 2 in, 2 out]
            n96 = call "Get SpinEcho Params.vi"("Spin Echo Parameters"="Spin Echo Parameters") -> ("max time"=w92:dbl, "min time"=w93:dbl, "# time points"=w94:i32, "# samples"=w95:i32, "Window Params Args"=w91:string)  [unwired: 6 in]
            n97 = control-ref of="Spin Echo contrast"() -> (w88:refnum<vi>)
            n98 = control-ref of="SpinEcho scans done"() -> (w86:refnum<vi>)
            n99 = call "Pulsed Experiment.vi"("Optimize Parameters"=w96, "Contrast XY Graph Refnum"=w88, "Experiment"=States."Spin Echo", "# samples"=w95, "# time points"=w94, "min time"=w93, "max time"=w92, "# scan iterations"="# SpinEcho scan iterations", "Window Parameters"=w91, "Save Contrast Options"="SpinEcho Save Options", "scans done ref"=w86) -> ()  [unwired: 5 in]
          }
          frame #1 {
            w99 = FALSE
            n100 = global write "Global Vars.vi" "SpinEcho-ing"(w99) -> ()
            n101 = property on="Spin Echo" class="Bool (strict)"("Value"=w99) -> ()  [unwired: 2 in, 2 out]
          }
        }
      }
      frame "CPMG" {
        n102 = flat-sequence {
          frame #0 {
            n103 = global write "Global Vars.vi" "CPMG-ing"(TRUE) -> ()
            n104 = property on="Optimize Parameters" class="Clust (strict)"() -> ("Value"=w100:T3)  [unwired: 2 in, 2 out]
            n105 = call "Get CPMG Params.vi"("CPMG Parameters"="CPMG Parameters") -> ("max time"=w111:dbl, "min time"=w110:dbl, "# time points"=w109:i32, "# samples"=w108:i32, "Window Params Args"=w107:string)  [unwired: 6 in]
            n106 = control-ref of="CPMG contrast"() -> (w103:refnum<vi>)
            n107 = control-ref of="CPMG scans done"() -> (w101:refnum<vi>)
            n108 = call "Pulsed Experiment.vi"("Optimize Parameters"=w100, "Contrast XY Graph Refnum"=w103, "Experiment"=States."CPMG", "# samples"=w108, "# time points"=w109, "min time"=w110, "max time"=w111, "# scan iterations"="# scan iterations", "Window Parameters"=w107, "Save Contrast Options"="Save CPMG Contrast Options", "scans done ref"=w101) -> ()  [unwired: 5 in]
          }
          frame #1 {
            w113 = FALSE
            n109 = global write "Global Vars.vi" "CPMG-ing"(w113) -> ()
            n110 = property on="CPMG" class="Bool (strict)"("Value"=w113) -> ()  [unwired: 2 in, 2 out]
          }
        }
      }
      frame "XY-4" {
        n111 = flat-sequence {
          frame #0 {
            n112 = global write "Global Vars.vi" "XY4-ing"(TRUE) -> ()
            n113 = property on="Optimize Parameters" class="Clust (strict)"() -> ("Value"=w119:T3)  [unwired: 2 in, 2 out]
            n114 = call "Get XY4 Params.vi"("XY-4 Parameters"="XY-4 Parameters") -> ("max time"=w121:dbl, "min time"=w122:dbl, "# time points"=w123:i32, "# samples"=w124:i32, "String"=w120:string)  [unwired: 6 in]
            n115 = control-ref of="XY-4 Normalized contrast"() -> (w115:refnum<vi>)
            n116 = call "Pulsed Experiment.vi"("Optimize Parameters"=w119, "Contrast XY Graph Refnum"=w115, "Experiment"=States."XY-4", "# samples"=w124, "# time points"=w123, "min time"=w122, "max time"=w121, "# scan iterations"="# scan iterations", "Window Parameters"=w120, "Save Contrast Options"="Save XY-4 Contrast Options") -> ()  [unwired: 6 in]
          }
          frame #1 {
            w126 = FALSE
            n117 = global write "Global Vars.vi" "XY4-ing"(w126) -> ()
            n118 = property on="XY-4" class="Bool (strict)"("Value"=w126) -> ()  [unwired: 2 in, 2 out]
          }
        }
      }
      frame "Exit" {
        w127 = FALSE
        n119 = global write "Global Vars.vi" "Scanning"(w127) -> ()
        n120 = global write "Global Vars.vi" "Counting"(w127) -> ()
        n121 = global write "Global Vars.vi" "Optimizing"(w127) -> ()
        n122 = property on="Count" class="Bool (strict)"("Value"=w127) -> ()  [unwired: 2 in, 2 out]
        n123 = property on="ESR" class="Bool (strict)"("Value"=w127) -> ()  [unwired: 2 in, 2 out]
        n124 = global write "Global Vars.vi" "ESR-ing"(w127) -> ()
        n125 = property on="Rabi" class="Bool (strict)"("Value"=w127) -> ()  [unwired: 2 in, 2 out]
        n126 = property on="Scan" class="Bool (strict)"("Value"=w127) -> ()  [unwired: 2 in, 2 out]
        n127 = property on="Spin Echo" class="Bool (strict)"("Value"=w127) -> ()  [unwired: 2 in, 2 out]
        n128 = property on="Optimize" class="Bool (strict)"("Value"=w127) -> ()  [unwired: 2 in, 2 out]
        n129 = global write "Global Vars.vi" "SpinEcho-ing"(w127) -> ()
        n130 = global write "Global Vars.vi" "Rabi-ing"(w127) -> ()
      }
      frame "Spectrum" {
      }
      frame "Stability" {
      }
    }
  }
  n131 = while {
    tunnel: w3 -> [w131]
    tunnel: w2 -> [w130]
    stop <- w129 stop-if-true
    n132 = event shown="[2] \"Count\": Value Change" {
      selector: _ -> [_ _ _ _ _ _ _ _ _ _ _ _ _ _ _ _]
      dyn-events: _ -> [_ _ _ _ _ _ _ _ _ _ _ _ _ _ _ _]
      timeout: _ -> [_ _ _ _ _ _ _ _ _ _ _ _ _ _ _ _]
      tunnel: w131 -> [w133 w140 w148 _ _ w166 w175 _ _ w186 w190 _ _ w207 w214 w222]
      tunnel: w130 -> [w132 w139 w147 _ _ w167 w174 _ _ w185 w189 _ _ w208 w213 w221]
      tunnel: [_ _ _ _ _ _ _ _ _ TRUE _ _ _ _ _ _] -> w129
      event "Scan": Value Change {
        n133 = event-data() -> ()  [unwired: 1 in, 5 out]
        n134 = case shown="False" "Scan" {
          tunnel: w133 -> [_ w137]
          tunnel: w132 -> [_ w136]
          frame False {
            n135 = global write "Global Vars.vi" "Scanning"(FALSE) -> ()
          }
          frame True {
            n136 = Enqueue Element(queue=w137, element=States."Scan", error in (no error)=w136) -> ()  [unwired: 1 in, 3 out]
          }
        }
      }
      event "Optimize": Value Change {
        n137 = event-data() -> ()  [unwired: 1 in, 5 out]
        n138 = case shown="True" "Optimize" {
          tunnel: w140 -> [_ w144]
          tunnel: w139 -> [_ w143]
          frame False {
          }
          frame True {
            n139 = global write "Global Vars.vi" "Counting"(FALSE) -> ()
            n140 = Enqueue Element(queue=w144, element=States."Optimize", error in (no error)=w143) -> ()  [unwired: 1 in, 3 out]
          }
        }
      }
      event "Count": Value Change {
        n141 = event-data() -> ()  [unwired: 1 in, 5 out]
        n142 = case shown="True" "Count" {
          tunnel: w148 -> [_ w151]
          tunnel: w147 -> [_ w150]
          frame False {
            n143 = global write "Global Vars.vi" "Counting"(FALSE) -> ()
          }
          frame True {
            n144 = global read "Global Vars.vi" "Pause SpinEcho"() -> (w155:bool)
            n145 = global read "Global Vars.vi" "Optimizing"() -> (w154:bool)
            n146 = global read "Global Vars.vi" "Pause Rabi"() -> (w156:bool)
            n147 = Or(x=w156, y=w155) -> (x .or. y?=w153:bool)
            n148 = Or(x=w154, y=w153) -> (x .or. y?=w152:bool)
            n149 = case shown="False" w152 {
              tunnel: w151 -> [w158 _]
              tunnel: w150 -> [w157 _]
              frame False {
                n150 = Enqueue Element(queue=w158, element=States."Count", error in (no error)=w157) -> ()  [unwired: 1 in, 3 out]
              }
              frame True {
                n151 = global write "Global Vars.vi" "Counting"(TRUE) -> ()
              }
            }
          }
        }
      }
      event "Counts Intensity Graph": Cursor Release {
        n152 = event-data() -> ("CursLoc"=w161:cluster{"X":dbl, "Y":dbl})  [unwired: 1 in, 7 out]
        n153 = flat-sequence {
          tunnel: w161 -> [w162]
          frame #0 {
            n154 = Unbundle By Name(w162) -> ("X"=w164:dbl, "Y"=w163:dbl)
            n155 = global write "Global Vars.vi" "X Pos"(w164) -> ()
            n156 = global write "Global Vars.vi" "Y Pos"(w163) -> ()
          }
          frame #1 {
            n157 = call "Update Position to Globals.vi"() -> ()  [unwired: 11 in, 1 out]
          }
        }
      }
      event "Z Voltage": Value Change {
        n158 = event-data() -> ()  [unwired: 1 in, 5 out]
        n159 = flat-sequence {
          frame #0 {
            n160 = global write "Global Vars.vi" "Z Pos"("Z Voltage") -> ()
          }
          frame #1 {
            n161 = call "Update Position to Globals.vi"() -> ()  [unwired: 11 in, 1 out]
          }
        }
      }
      event "ESR": Value Change {
        n162 = event-data() -> ()  [unwired: 1 in, 5 out]
        n163 = case shown="True" "ESR" {
          tunnel: w166 -> [_ w171]
          tunnel: w167 -> [_ w170]
          frame False {
            n164 = global write "Global Vars.vi" "ESR-ing"(FALSE) -> ()
          }
          frame True {
            n165 = Enqueue Element(queue=w171, element=States."ESR", error in (no error)=w170) -> ()  [unwired: 1 in, 3 out]
          }
        }
      }
      event "Green Laser", "Microwave", "Green Laser (low-T)": Value Change {
        n166 = event-data() -> ()  [unwired: 1 in, 5 out]
        n167 = Enqueue Element(queue=w175, element=States."Hold", error in (no error)=w174) -> ()  [unwired: 1 in, 3 out]
      }
      event Timeout {
        n168 = event-data() -> ()  [unwired: 1 in, 2 out]
      }
      event "Z AO Channel", "Y AO Channel", "Counter(s)", "Sample clock line", "spinapi.dll", "HoldChannel.exe", "Laser voltage", "X AO Channel": Value Change {
        n169 = event-data() -> ()  [unwired: 1 in, 5 out]
        n170 = global write "Channels.vi" "Laser voltage"("Laser voltage") -> ()
        n171 = global write "Channels.vi" "X Channel"("X AO Channel") -> ()
        n172 = global write "Channels.vi" "Y Channel"("Y AO Channel") -> ()
        n173 = global write "Channels.vi" "Counter(s)"("Counter(s)") -> ()
        n174 = global write "Channels.vi" "Sample clock line"("Sample clock line") -> ()
        n175 = global write "Channels.vi" "HoldChannel.exe"("HoldChannel.exe") -> ()
        n176 = global write "Channels.vi" "spinapi.dll"("spinapi.dll") -> ()
        n177 = global write "Channels.vi" "Z Channel"("Z AO Channel") -> ()
      }
      event Panel Close? {
        w184 = FALSE
        n178 = event-data() -> ()  [unwired: 1 in, 3 out]
        n179 = Enqueue Element(queue=w186, element=States."Exit", error in (no error)=w185) -> ()  [unwired: 1 in, 3 out]
        n180 = global write "Global Vars.vi" "Optimizing"(w184) -> ()
        n181 = global write "Global Vars.vi" "Scanning"(w184) -> ()
        n182 = global write "Global Vars.vi" "Counting"(w184) -> ()
        n183 = global write "Global Vars.vi" "ESR-ing"(w184) -> ()
        n184 = event-data() -> ()  [unwired: 2 in, 1 out]
      }
      event "Rabi": Value Change {
        n185 = event-data() -> ()  [unwired: 1 in, 5 out]
        n186 = case shown="False" "Rabi" {
          tunnel: w190 -> [_ w194]
          tunnel: w189 -> [_ w193]
          frame False {
            n187 = global write "Global Vars.vi" "Rabi-ing"(FALSE) -> ()
          }
          frame True {
            n188 = Enqueue Element(queue=w194, element=States."Rabi", error in (no error)=w193) -> ()  [unwired: 1 in, 3 out]
          }
        }
      }
      event "Rabi Pause": Value Change {
        n189 = event-data() -> ()  [unwired: 1 in, 5 out]
        n190 = case shown="False" "Rabi Pause" {
          frame False {
            n191 = while {
              stop <- w198 continue-if-true
              n192 = property on="Count" class="Bool (strict)"() -> ("Value"=w198:bool)  [unwired: 2 in, 2 out]
              n193 = case shown="False" w198 {
                frame False {
                  n194 = global write "Global Vars.vi" "Pause Rabi"(FALSE) -> ()
                }
                frame True {
                }
              }
            }
            n195 = global write "Global Vars.vi" "Counting"(FALSE) -> ()
          }
          frame True {
            n196 = global write "Global Vars.vi" "Pause Rabi"(TRUE) -> ()
          }
        }
      }
      event "Pause Spin Echo": Value Change {
        n197 = event-data() -> ()  [unwired: 1 in, 5 out]
        n198 = case shown="False" "Pause Spin Echo" {
          frame False {
            n199 = while {
              stop <- w203 continue-if-true
              n200 = property on="Count" class="Bool (strict)"() -> ("Value"=w203:bool)  [unwired: 2 in, 2 out]
              n201 = case shown="False" w203 {
                frame False {
                  n202 = global write "Global Vars.vi" "Pause SpinEcho"(FALSE) -> ()
                }
                frame True {
                }
              }
            }
            n203 = global write "Global Vars.vi" "Counting"(FALSE) -> ()
          }
          frame True {
            n204 = global write "Global Vars.vi" "Pause SpinEcho"(TRUE) -> ()
          }
        }
      }
      event "Spin Echo": Value Change {
        n205 = event-data() -> ()  [unwired: 1 in, 5 out]
        n206 = case shown="True" "Spin Echo" {
          tunnel: w207 -> [_ w211]
          tunnel: w208 -> [_ w210]
          frame False {
            n207 = global write "Global Vars.vi" "SpinEcho-ing"(FALSE) -> ()
          }
          frame True {
            n208 = Enqueue Element(queue=w211, element=States."Spin Echo", error in (no error)=w210) -> ()  [unwired: 1 in, 3 out]
          }
        }
      }
      event "CPMG": Value Change {
        n209 = event-data() -> ()  [unwired: 1 in, 5 out]
        n210 = case shown="True" "CPMG" {
          tunnel: w214 -> [_ w218]
          tunnel: w213 -> [_ w217]
          frame False {
            n211 = global write "Global Vars.vi" "CPMG-ing"(FALSE) -> ()
          }
          frame True {
            n212 = Enqueue Element(queue=w218, element=States."CPMG", error in (no error)=w217) -> ()  [unwired: 1 in, 3 out]
          }
        }
      }
      event "XY-4": Value Change {
        n213 = event-data() -> ()  [unwired: 1 in, 5 out]
        n214 = case shown="True" "XY-4" {
          tunnel: w222 -> [_ w225]
          tunnel: w221 -> [_ w224]
          frame False {
            n215 = global write "Global Vars.vi" "XY4-ing"(FALSE) -> ()
          }
          frame True {
            n216 = Enqueue Element(queue=w225, element=States."XY-4", error in (no error)=w224) -> ()  [unwired: 1 in, 3 out]
          }
        }
      }
    }
  }
  n217 = while {
    stop <- FALSE stop-if-true
    n218 = global read "Global Vars.vi" "Counting"() -> (w228:bool)
    n219 = case shown="True" w228 {
      frame False {
      }
      frame True {
        n220 = global read "Global Vars.vi" "Optimizing"() -> (w230:bool)
        n221 = case shown="False" w230 {
          frame False {
            n222 = global read "Global Vars.vi" "Pause SpinEcho"() -> (w232:bool)
            n223 = global read "Global Vars.vi" "Pause Rabi"() -> (w233:bool)
            n224 = Or(x=w233, y=w232) -> (x .or. y?=w231:bool)
            n225 = case shown="True" w231 {
              frame False {
              }
              frame True {
                n226 = flat-sequence {
                  frame #0 {
                    n227 = control-ref of="Counts Chart"() -> (w234:refnum<vi>)
                    n228 = control-ref of="Counts/s"() -> (w235:refnum<vi>)
                    n229 = call "Counter.vi"("Counts Chart Refnum"=w234, "Counts/s Ref"=w235) -> ()  [unwired: 10 in]
                  }
                  frame #1 {
                    n230 = property on="Count" class="Bool (strict)"("Value"=FALSE) -> ()  [unwired: 2 in, 2 out]
                  }
                }
              }
            }
          }
          frame True {
            n231 = while {
              stop <- w239 stop-if-true
              n232 = global read "Global Vars.vi" "Counts"() -> (w237:u32)
              n233 = property on="Counts Chart" class="WFChart (strict)"("Value"=w237) -> ()  [unwired: 2 in, 2 out]
              n234 = property on="Counts/s" class="DigNum (strict)"("Value"=w237) -> ()  [unwired: 2 in, 2 out]
              n235 = global read "Global Vars.vi" "Counting"() -> (w240:bool)
              n236 = Not(x=w240) -> (.not. x?=w239:bool)
              n237 = Wait (ms)(milliseconds to wait=100) -> ()  [unwired: 1 out]
            }
          }
        }
      }
    }
    n238 = Wait (ms)(milliseconds to wait=100) -> ()  [unwired: 1 out]
  }
